vi "SubVI.vi"(8 "error in (no error)":errorcluster) -> (0 "error out":errorcluster)   [LabVIEW 2013]
panel:
  out "Loop":i32
  in  "Exit":bool
  # "§Ú¬O¡@¢á¢ã¢Ð¡@¢ä¢×"
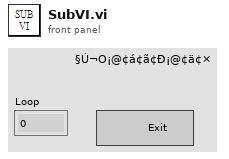
[diagram p1: front panel]
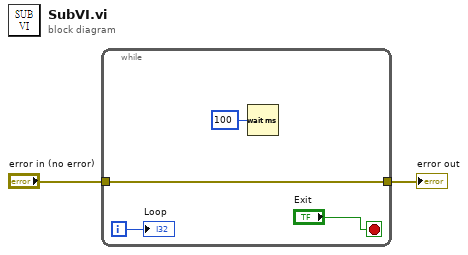
[diagram p0: block diagram]
diagram:
  n1 = while {
    tunnel: [w4] -> w2
    tunnel: "error in (no error)" -> [w4]
    i -> [w3]
    stop <- "Exit" stop-if-true
    n2 = Wait (ms)(milliseconds to wait=u32 100) -> ()  [unwired: 1 out]
    "Loop" <- w3
  }
  "error out" <- w2
